vi "8.vi"() -> ()   [LabVIEW 2020]
panel:
  out "Number 2":dbl
  in  "Power":dbl
  in  "Number":dbl
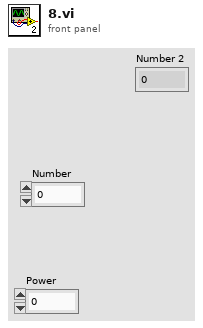
[diagram p1: front panel]
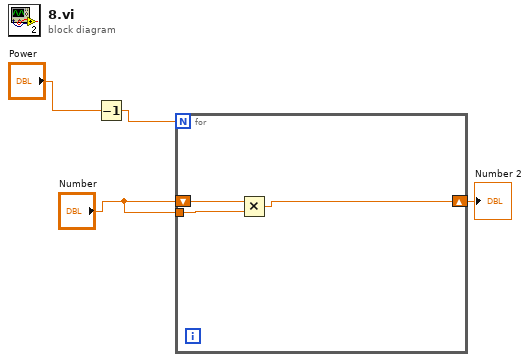
[diagram p0: block diagram]
diagram:
  n1 = Decrement(x="Power") -> (x-1=w1:dbl)
  n2 = for {
    N: w1 -> [_]
    shift-right: [w6] -> w3
    shift-left: "Number" -> [w7]
    tunnel: "Number" -> [w5]
    n3 = Multiply(x=w7, y=w5) -> (x*y=w6:dbl)
  }
  "Number 2" <- w3
